vi "User-defined Gate.vi"() -> ()   [LabVIEW 2019]
uses:
  Graphs/XY Graph/XY Plot Data.ctl
panel:
  in  "User-defined Gate":T1
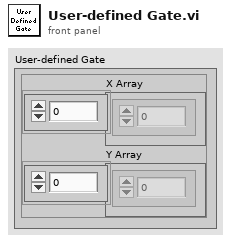
[diagram p1: front panel]
types:
  T1 = typedef "XY Plot Data.ctl" = cluster{"X Array":dbl[], "Y Array":dbl[]}
diagram:
